vi "ArmIncrementLE.vi"(9 "AddE":dbl, 10 "AddL":dbl) -> ()   [LabVIEW 2020]
doc: "Increment Rotate, Lift, Extend values\n\nInput:\n--AddR--Double--how much to increment Rotate\n--AddL--Double--how much to increment Lift\n--AddE--Double--how much to increment Extend"
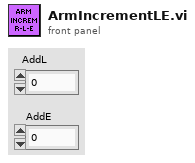
[diagram p1: front panel]
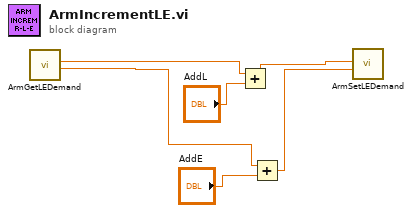
[diagram p0: block diagram]
diagram:
  n1 = call "ArmGetLEDemand.vi"() -> ("ExtendPositonDemand(in)"=w1:dbl, "LiftPositionDemand(d)"=w2:dbl)  [unwired: 10 in]
  n2 = Add(x=w2, y="AddL") -> (x+y=w4:dbl)
  n3 = Add(x=w1, y="AddE") -> (x+y=w3:dbl)
  n4 = call "ArmSetLEDemand.vi"("SetExtendPositonDemand(in)"=w3, "SetLIftPostionDemand(d)"=w4) -> ()  [unwired: 10 in]
